vi "PID Controller.vi"(6 "reinitialize? (F)":bool, 7 "output range":cluster{"high":dbl, "low":dbl}={"high"=100.0, "low"=-100.0} {"low" format="%.2f"; "high" format="%.2f"}, 8 "dt (s)":dbl=0.02 format="%.3f", 9 "PID gains":T1={"proportional gain (Kp)"=1.0, "integral gain (Ki)"=0.0, "derivative gain (Kd)"=0.0} {"derivative gain (Kd)" format="%.3f"; "integral gain (Ki)" format="%.3f"; "proportional gain (Kp)" format="%.3f"}, 10 "process variable":dbl format="%.2f", 11 "setpoint":dbl format="%.2f") -> (1 "Err/Out Chart":cluster{dbl, dbl}(graph), 2 "SP/PV Chart":cluster{"setpoint":dbl, "process variable":dbl}(graph), 3 "output":dbl format="%.2f")   [LabVIEW 2023]
panel:
  in  "advanced":cluster{"alpha":dbl, "i-zone":dbl}={"alpha"=nan, "i-zone"=nan} {"i-zone" format="%.2f"; "alpha" format="%.2f"}
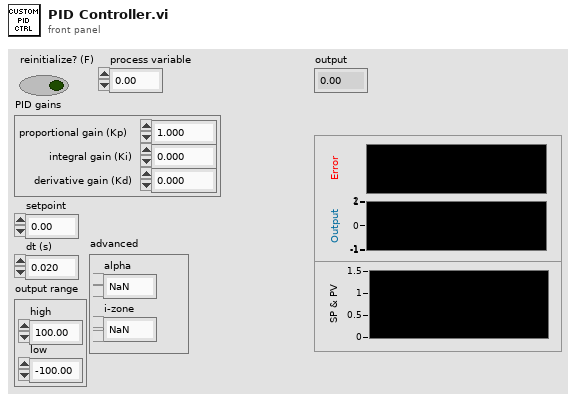
[diagram p1: front panel]
types:
  T1 = cluster{"proportional gain (Kp)":dbl, "integral gain (Ki)":dbl, "derivative gain (Kd)":dbl}
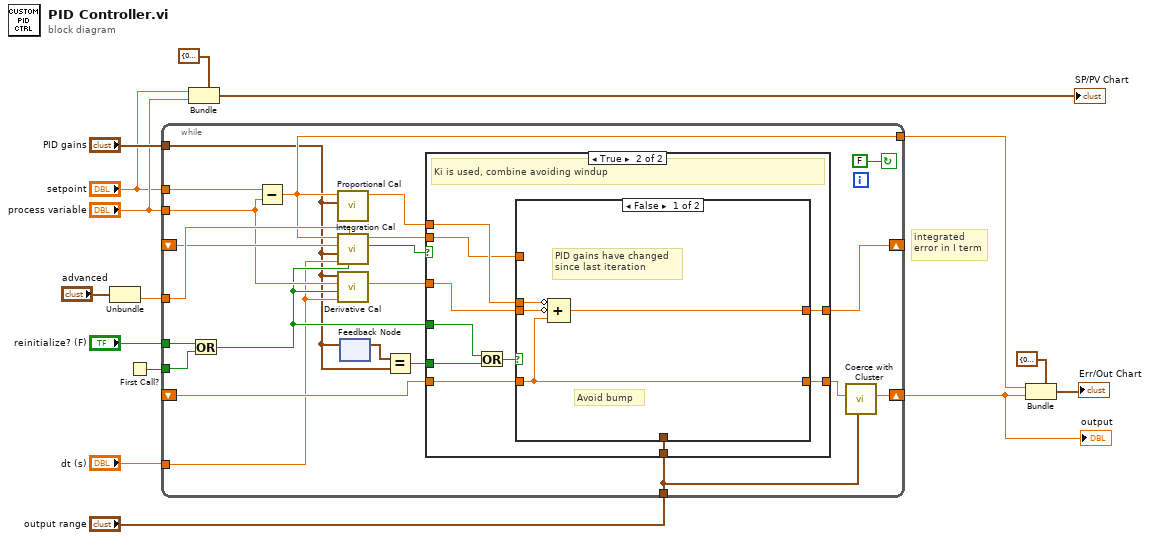
[diagram p0: block diagram]
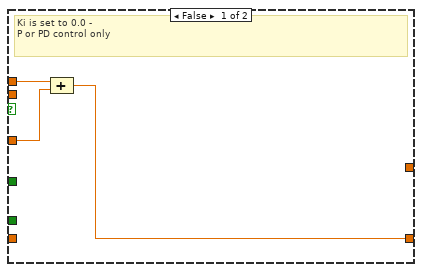
[diagram p2: hidden frame]
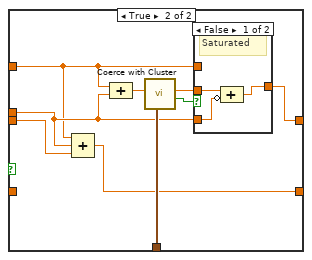
[diagram p3: hidden frame]
diagram:
  # "integrated\nerror in I term"
  n1 = Unbundle("advanced") -> ("i-zone"=w1:dbl)  [unwired: 1 out]
  n2 = First Call?() -> (First Call?: T/F=w14:bool)
  n3 = while {
    tunnel: "dt (s)" -> [w17]
    tunnel: "process variable" -> [w19]
    shift-right: [w31] -> w4
    shift-left: _ -> [w37]
    shift-right: [w36] -> _
    shift-left: _ -> [w22]
    tunnel: w14 -> [w29]
    tunnel: "PID gains" -> [w16]
    tunnel: "output range" -> [w33]
    tunnel: "setpoint" -> [w30]
    tunnel: "reinitialize? (F)" -> [w28]
    tunnel: [w21] -> w3
    tunnel: w1 -> [w25]
    stop <- FALSE continue-if-true
    n4 = Or(x=w28, y=w29) -> (x .or. y?=w18:bool)
    n5 = Subtract(x=w30, y=w19) -> (x-y=w21:dbl)
    n6 = call "Proportional Cal.vi"("PID gains"=w16, "Error"=w21) -> ("Proportional Term"=w26:dbl)  [unwired: 9 in]
    n7 = call "Integration Cal.vi"("Reinit"=w18, "i-zone"=w25, "dT"=w17, "PID gains"=w16, "Integration Error"=w22, "Curr Error"=w21) -> ("Integral Used"=w23:bool, "Integral Term"=w24:dbl)  [unwired: 4 in]
    n8 = call "Derivative Cal.vi"("dt"=w17, "Reinit"=w18, "process variable in"=w19, "PID gains"=w16) -> ("deriv Term"=w20:dbl)  [unwired: 7 in]
    n9 = feedback #1() -> (w27:T1)  [unwired: 1 in]
    n10 = feedback-in #1(w16) -> ()
    n11 = Equal?(x=w27, y=w16) -> (x = y?=w34:bool)
    n12 = case shown="True" w23 {
      tunnel: [_ w47] -> w36
      tunnel: w37 -> [_ w48]
      tunnel: w20 -> [w38 w46]
      tunnel: w18 -> [_ w45]
      tunnel: w34 -> [_ w44]
      tunnel: w33 -> [_ w43]
      tunnel: w24 -> [_ w42]
      tunnel: [w39 w41] -> w32
      tunnel: w26 -> [w40 w50]
      frame False {
        # "Ki is set to 0.0 -\nP or PD control only"
        n13 = Compound Arithmetic op=ADD(w40, w38) -> (w39:dbl)
      }
      frame True {
        # "Ki is used, combine avoiding windup"
        n14 = Or(x=w45, y=w44) -> (x .or. y?=w49:bool)
        n15 = case shown="False" w49 {
          tunnel: w42 -> [_ w55]
          tunnel: w50 -> [w54 w56]
          tunnel: w48 -> [w51 _]
          tunnel: [w52 w63] -> w47
          tunnel: w46 -> [w53 w58]
          tunnel: w43 -> [_ w59]
          tunnel: [w51 w57] -> w41
          frame False {
            # "Avoid bump"
            # "PID gains have changed\nsince last iteration"
            n16 = Compound Arithmetic op=ADD(invert w54, invert w53, w51) -> (w52:dbl)
          }
          frame True {
            n17 = Compound Arithmetic op=ADD(w55, w56, w58) -> (w57:dbl)
            n18 = Compound Arithmetic op=ADD(w55, w56) -> (w60:dbl)
            n19 = call <vilib>:"Coerce with Cluster.vi"("value in"=w60, "output range"=w59) -> ("coerced value"=w61:dbl, "In Range?"=w62:bool)  [unwired: 7 in]
            n20 = case shown="False" w62 {
              tunnel: w55 -> [_ w67]
              tunnel: [w64 w67] -> w63
              tunnel: w61 -> [w66 _]
              tunnel: w56 -> [w65 _]
              frame False {
                # "Saturated"
                n21 = Compound Arithmetic op=ADD(w66, invert w65) -> (w64:dbl)
              }
              frame True {
                # "! Saturated"
              }
            }
          }
        }
      }
    }
    n22 = call <vilib>:"Coerce with Cluster.vi"("value in"=w32, "output range"=w33) -> ("coerced value"=w31:dbl)  [unwired: 7 in, 1 out]
  }
  "output" <- w4
  n23 = Bundle(cluster=cluster{"setpoint":dbl, "process variable":dbl} {"setpoint"=0.0, "process variable"=0.0}, "setpoint"="setpoint", "process variable"="process variable") -> (→"SP/PV Chart":cluster{"setpoint":dbl, "process variable":dbl})
  n24 = Bundle(cluster=cluster{"Error":dbl, "Output":dbl} {"Error"=0.0, "Output"=0.0}, "Error"=w3, "Output"=w4) -> (→"Err/Out Chart":cluster{"Error":dbl, "Output":dbl})
